vi "PH_Beamline_Common.set Double Filter.vi"(1 "Alignment (vertical)":T1=enum."vertical", 2 "CtlRef":refnum<vi>, 3 "State":i16, 4 "no link":bool, 5 "error in (no error)":errorcluster) -> (19 "error out":errorcluster)   [LabVIEW 2014, in "PH_Beamline_Common.lvlib"]
uses:
  PH_Beamline_Common.lvlib
  PH_Common/Picture/PH_Picture.Alignment.ctl
  PH_Common/PH_Common.lvlib
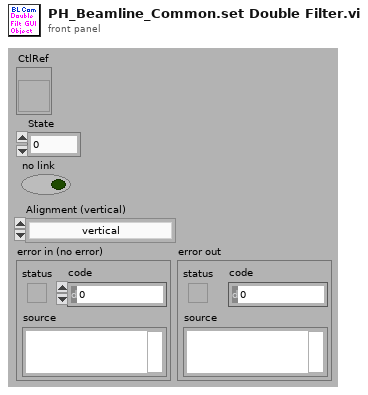
[diagram p1: front panel]
types:
  T1 = typedef "PH_Common.lvlib/PH_Picture.Alignment.ctl" = enum16{"neutral", "left", "right", "up", "down", "vertical", "horizontal", "left down to right up", "left up to right down"}
  T2 = cluster{"left":i16, "top":i16, "right":i16, "bottom":i16}[]
  T3 = cluster{"left":i16, "top":i16, "right":i16, "bottom":i16}
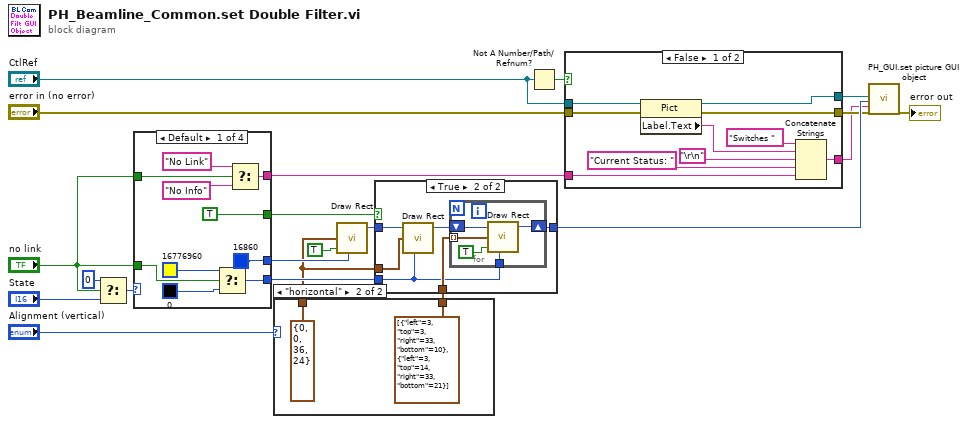
[diagram p0: block diagram]
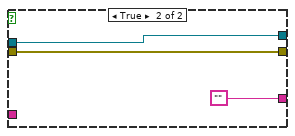
[diagram p2: hidden frame]
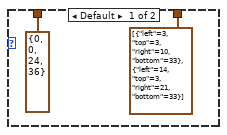
[diagram p3: hidden frame]
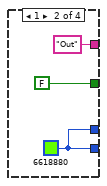
[diagram p5: hidden frame]
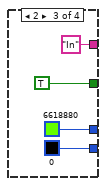
[diagram p6: hidden frame]
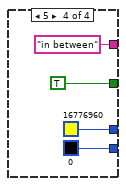
[diagram p7: hidden frame]
diagram:
  n1 = Select(t=i16 0, s="no link", f="State") -> (s? t:f=w18:i16)
  n2 = case shown="Default" w18 {
    tunnel: "no link" -> [w29 _ _ _]
    tunnel: [u32 16860 w34 u32 6618880 u32 16776960] -> w16
    tunnel: [w26 w34 u32 0 u32 0] -> w12
    tunnel: [TRUE FALSE TRUE TRUE] -> w10
    tunnel: "no link" -> [w23 _ _ _]
    tunnel: [w22 "Out" "In" "in between"] -> w1
    frame Default {
      n3 = Select(t=u32 16776960, s=w29, f=u32 0) -> (s? t:f=w26:u32)
      n4 = Select(t="No Link", s=w23, f="No Info") -> (s? t:f=w22:string)
    }
    frame 1 {
      w34 = u32 6618880
    }
    frame 2 {
    }
    frame 5 {
    }
  }
  n5 = case shown="\"horizontal\"" "Alignment (vertical)" {
    tunnel: [T2 [{"left"=3, "top"=3, "right"=10, "bottom"=33}, {"left"=14, "top"=3, "right"=21, "bottom"=33}] T2 [{"left"=3, "top"=3, "right"=33, "bottom"=10}, {"left"=3, "top"=14, "right"=33, "bottom"=21}]] -> w14
    tunnel: [T3 {"left"=0, "top"=0, "right"=24, "bottom"=36} ("rect") T3 {"left"=0, "top"=0, "right"=36, "bottom"=24} ("rect")] -> w11
    frame Default {
    }
    frame "horizontal" {
    }
  }
  n6 = call <vilib>:"Draw Rect.vi"("rect"=w11, "fill?(F)"=TRUE, "color(black)"=w16) -> ("new picture"=w13:picture)  [unwired: 6 in]
  n7 = case shown="True" w10 {
    tunnel: [w47 w53] -> w15
    tunnel: w14 -> [_ w52]
    tunnel: w13 -> [w47 w51]
    tunnel: w12 -> [_ w49]
    tunnel: w11 -> [_ w48]
    frame False {
    }
    frame True {
      n8 = call <vilib>:"Draw Rect.vi"("picture"=w51, "rect"=w48, "color(black)"=w49) -> ("new picture"=w50:picture)  [unwired: 6 in]
      n9 = for {
        tunnel: w49 -> [w57]
        tunnel: w52 -> [w55] mode=indexing
        shift-right: [w58] -> w53
        shift-left: w50 -> [w56]
        n10 = call <vilib>:"Draw Rect.vi"("picture"=w56, "rect"=w55, "fill?(F)"=TRUE, "color(black)"=w57) -> ("new picture"=w58:picture)  [unwired: 5 in]
      }
    }
  }
  n11 = Not A Number/Path/Refnum?(number/path/refnum="CtlRef") -> (NaN/Path/Refnum?=w8:bool)
  n12 = case shown="False" w8 {
    tunnel: "CtlRef" -> [w64 w71]
    tunnel: "error in (no error)" -> [w63 w70]
    tunnel: w1 -> [w62 _]
    tunnel: [w61 w71] -> w4
    tunnel: [w60 w70] -> w6
    tunnel: [w59 ""] -> w3
    frame False {
      n13 = property class="Pict"(reference=w64, error in=w63) -> (reference out=w61:refnum<vi>, error out=w60:errorcluster, "Label.Text"=w67:string)
      n14 = Concatenate Strings("Switches " ("string"), w67, "\r\n", "Current Status: " ("string"), w62) -> (w59:string)
    }
    frame True {
    }
  }
  n15 = call "PH_GUI.set picture GUI object.vi"("CtlRef"=w4, "Picture"=w15, "Tip Strip (\"\")"=w3, "error in (no error)"=w6) -> ("error out"=→"error out":errorcluster)  [unwired: 15 in]
